vi "Logging.vi"(8 "error in (no error)":errorcluster, 11 "Node Ptr":T2 format="%.0x") -> (0 "error out":errorcluster)   [LabVIEW 2020, in "AIM MIL-STD-1553 System Explorer.lvlib" / "Implementation.lvlib"]
uses:
  Implementation.lvlib
  <vilib>/NI VeriStand/Custom Device API/Custom Device API.lvlib
  Scripting/AIM MIL-STD-1553 Scripting.lvlib
  <vilib>/NI VeriStand/Custom Device API/Custom Device Item Ref.ctl
  Shared/Data Word Format.ctl
panel:
  in  "Data Word Format":T1
  in  "Timestamp Filename":bool
  in  "File Name":string
  out "Example Log File Path":string
  in  "Enable Logging":bool
  in  "Log Directory":string
  in  "SHDocVw.IWebBrowser":refnum<k7>(container)
  in  "General Header":cluster{"Section Name":string}={"Section Name"="MIL-STD-1553 - Logging"}
  in  "Description":string
  out "Name":string
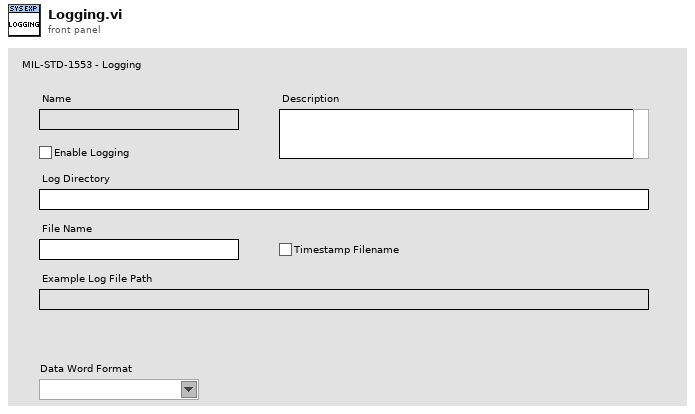
[diagram p1: front panel]
types:
  T1 = typedef "Data Word Format.ctl" = string
  T2 = typedef "Custom Device API.lvlib/Custom Device Item Ref.ctl" = u64
  T3 = typedef "Custom Device API.lvlib/Custom Device Item Info.ctl" = cluster{"Name":string, "Is Channel":bool, "GUID":string, "Is Waveform":bool}
  T4 = typedef "Custom Device API.lvlib/Custom Device Commands.ctl" = enum16{"Default", "Item renamed", "Shutdown", "Dynamic button pressed"}
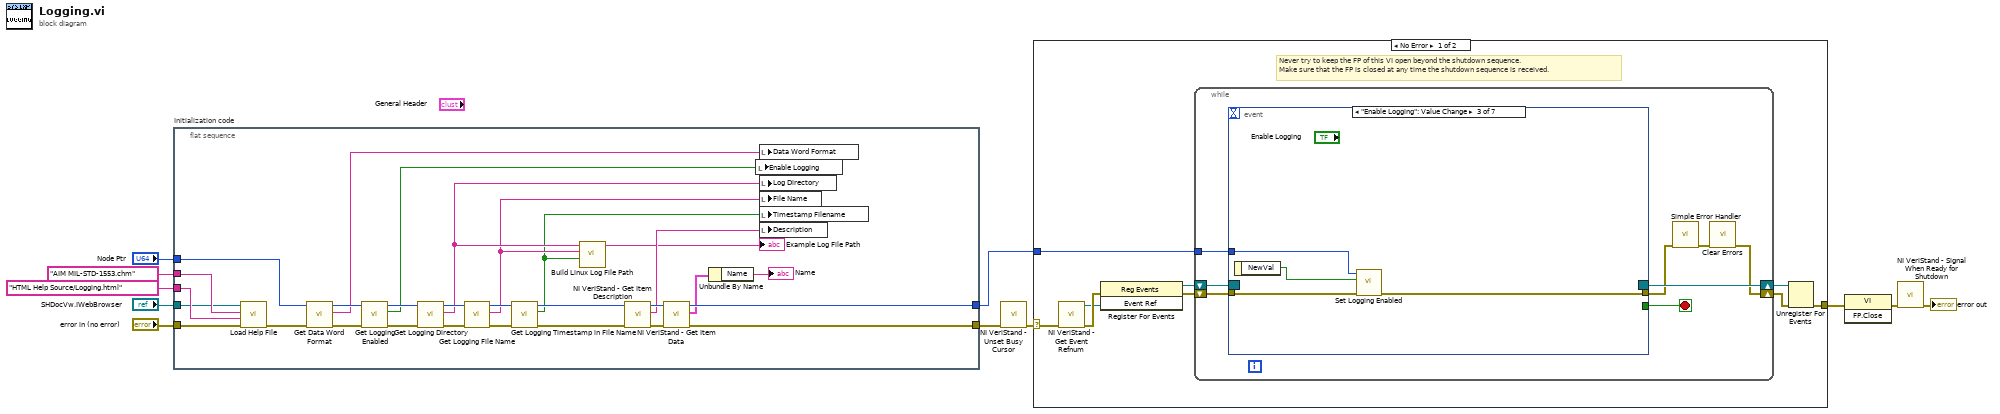
[diagram p0: block diagram]
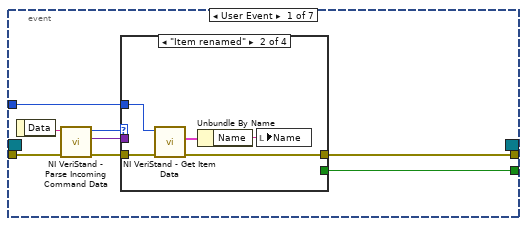
[diagram p2: hidden frame]
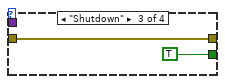
[diagram p4: hidden frame]
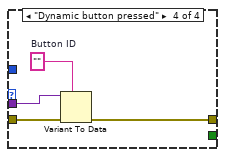
[diagram p5: hidden frame]
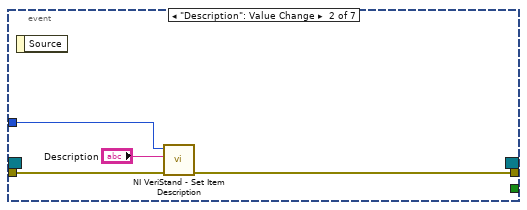
[diagram p6: hidden frame]
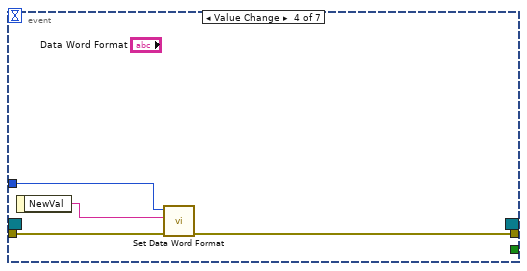
[diagram p7: hidden frame]
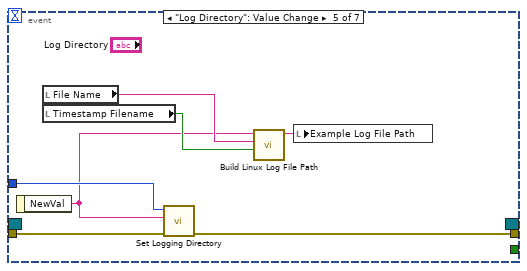
[diagram p8: hidden frame]
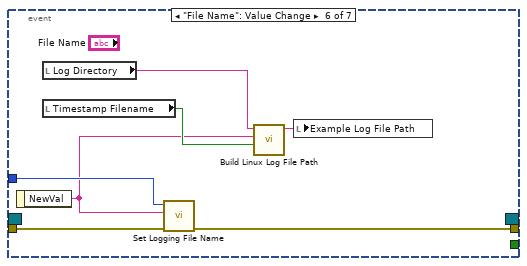
[diagram p9: hidden frame]
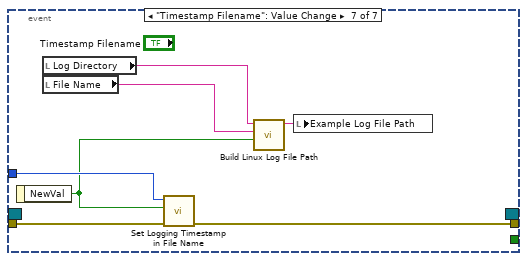
[diagram p10: hidden frame]
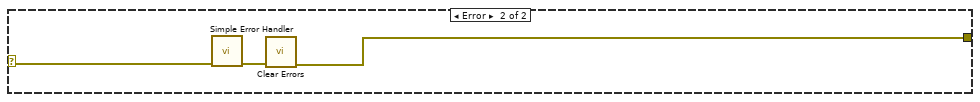
[diagram p11: hidden frame]
diagram:
  n1 = flat-sequence "Initialization code" {
    tunnel: "error in (no error)" -> [w34]
    tunnel: "Node Ptr" -> [w24]
    tunnel: [w36] -> w7
    tunnel: [w40] -> w4
    tunnel: "SHDocVw.IWebBrowser" -> [w31]
    tunnel: "HTML Help Source/Logging.html" ("CD_CHM_Section") -> [w33]
    tunnel: "AIM MIL-STD-1553.chm" ("CD_CHM_FileName") -> [w32]
    frame #0 {
      n2 = call "Load Help File.vi"("error in (no error)"=w34, "HTML File to Load"=w33, "Main CHM File"=w32, "Browser"=w31) -> ("error out"=w29:errorcluster)  [unwired: 7 in]
      n3 = call "Get Data Word Format.vi"("error in"=w29, "logging section"=w24) -> ("error out"=w25:errorcluster, "data word format"=w22:T1, "logging section out"=w23:T2)  [unwired: 7 in]
      n4 = call "Get Logging Enabled.vi"("error in"=w25, "logging section"=w23) -> ("error out"=w28:errorcluster, "logging enabled"=w26:bool, "logging section out"=w27:T2)  [unwired: 7 in]
      n5 = call "Get Logging Directory.vi"("error in"=w28, "logging section"=w27) -> ("error out"=w20:errorcluster, "directory"=w14:string, "logging section out"=w21:T2)  [unwired: 7 in]
      n6 = call "Get Logging File Name.vi"("error in"=w20, "logging section"=w21) -> ("error out"=w19:errorcluster, "file name"=w13:string, "logging section out"=w18:T2)  [unwired: 7 in]
      n7 = call "Get Logging Timestamp in File Name.vi"("error in"=w19, "logging section"=w18) -> ("error out"=w17:errorcluster, "timestamp in file name"=w12:bool, "logging section out"=w16:T2)  [unwired: 7 in]
      n8 = call "Build Linux Log File Path.vi"("Timestamp"=w12, "Name"=w13, "Log File Directory"=w14) -> ("Log File Path"=→"Example Log File Path":string)  [unwired: 7 in, 1 out]
      n9 = call <vilib>:"NI VeriStand - Get Item Description.vi"("error in (no error)"=w17, "Item Ref in"=w16) -> ("error out"=w38:errorcluster, "Description"=w35:string, "Item Ref out"=w39:T2)  [unwired: 7 out]
      n10 = call <vilib>:"NI VeriStand - Get Item Data.vi"("error in (no error)"=w38, "Item Ref in"=w39) -> ("error out"=w36:errorcluster, "Item Info"=w37:T3, "Item Ref out"=w40:T2)  [unwired: 7 out]
      n11 = Unbundle By Name(w37) -> ("Name"=→"Name":string)
      n12 = local write "Enable Logging"(w26) -> ()
      n13 = local write "Data Word Format"(w22) -> ()
      n14 = local write "Log Directory"(w14) -> ()
      n15 = local write "File Name"(w13) -> ()
      n16 = local write "Timestamp Filename"(w12) -> ()
      n17 = local write "Description"(w35) -> ()
    }
  }
  n18 = call <vilib>:"NI VeriStand - Unset Busy Cursor.vi"("error in (no error)"=w7) -> ("error out"=w6:errorcluster)  [unwired: 10 out]
  n19 = case shown="No Error" w6 {
    selector: w6 -> [w41 w113]
    tunnel: [w46 w111] -> w11
    tunnel: w4 -> [w42 _]
    frame No Error {
      # "Never try to keep the FP of this VI open beyond the shutdown sequence.\nMake sure that the FP is closed at any time the shutdown sequence is received."
      n20 = call <vilib>:"NI VeriStand - Get Event Refnum.vi"("error in (no error)"=w41) -> ("error out"=w49:errorcluster, "Event Ref"=w45:refnum<user-event>)  [unwired: 9 out]
      n21 = register-events(error in=w49, w45) -> (reference out=w43:refnum<event-registration>, error out=w44:errorcluster)  [unwired: 1 in]
      n22 = while {
        tunnel: w42 -> [w53]
        shift-right: [w50] -> w47
        shift-left: w44 -> [w56]
        shift-right: [w57] -> w48
        shift-left: w43 -> [w55]
        stop <- w54 stop-if-true
        n23 = event shown="[2] \"Enable Logging\": Value Change" {
          selector: w55 -> [_ _ _ _ _ _ _]
          dyn-events: [_ _ _ _ _ _ _] -> w57
          timeout: _ -> [_ _ _ _ _ _ _]
          tunnel: w56 -> [w65 w80 w85 w88 w96 w103 w110]
          tunnel: [w61 _ _ _ _ _ _] -> w54
          tunnel: [w60 w79 w84 w89 w94 w102 w109] -> w52
          tunnel: w53 -> [w59 w81 w83 w87 w95 w101 w108]
          event User Event {
            n24 = event-data() -> ("Data"=w64:string)  [unwired: 1 out]
            n25 = call <vilib>:"NI VeriStand - Parse Incoming Command Data.vi"("error in (no error)"=w65, "Incoming data"=w64) -> ("error out"=w63:errorcluster, "Outgoing data"=w58:variant, "Action"=w62:T4)  [unwired: 7 out]
            n26 = case shown="\"Item renamed\"" w62 {
              tunnel: w63 -> [w66 w71 w72 w77]
              tunnel: [_ _ TRUE _] -> w61
              tunnel: [w66 w68 w72 w74] -> w60
              tunnel: w59 -> [_ w70 _ _]
              tunnel: w58 -> [_ _ _ w76]
              frame "Default", Default {
              }
              frame "Item renamed" {
                n27 = call <vilib>:"NI VeriStand - Get Item Data.vi"("error in (no error)"=w71, "Item Ref in"=w70) -> ("error out"=w68:errorcluster, "Item Info"=w69:T3)  [unwired: 8 out]
                n28 = Unbundle By Name(w69) -> ("Name"=w67:string)
                n29 = local write "Name"(w67) -> ()
              }
              frame "Shutdown" {
              }
              frame "Dynamic button pressed" {
                w75 = ""  # Button ID
                n30 = Variant To Data(error in=w77, type=w75, Variant=w76) -> (error out=w74:errorcluster)  [unwired: 1 out]
              }
            }
          }
          event "Description": Value Change {
            n31 = event-data() -> ()  [unwired: 2 out]
            n32 = call <vilib>:"NI VeriStand - Set Item Description.vi"("error in (no error)"=w80, "Description"="Description", "Item Ref in"=w81) -> ("error out"=w79:errorcluster)  [unwired: 8 out]
          }
          event "Enable Logging": Value Change {
            n33 = event-data() -> ("NewVal"=w82:bool)  [unwired: 1 out]
            n34 = call "Set Logging Enabled.vi"("error in"=w85, "logging enabled"=w82, "logging section"=w83) -> ("error out"=w84:errorcluster)  [unwired: 7 in, 1 out]
          }
          event Value Change {
            n35 = event-data() -> ("NewVal"=w86:T1)  [unwired: 1 out]
            n36 = call "Set Data Word Format.vi"("error in"=w88, "data word format"=w86, "logging section"=w87) -> ("error out"=w89:errorcluster)  [unwired: 7 in, 1 out]
          }
          event "Log Directory": Value Change {
            n37 = event-data() -> ("NewVal"=w90:string)  [unwired: 1 out]
            n38 = local read "File Name"() -> (w92:string)
            n39 = local read "Timestamp Filename"() -> (w91:bool)
            n40 = call "Set Logging Directory.vi"("error in"=w96, "directory"=w90, "logging section"=w95) -> ("error out"=w94:errorcluster)  [unwired: 6 in, 1 out]
            n41 = call "Build Linux Log File Path.vi"("Timestamp"=w91, "Name"=w92, "Log File Directory"=w90) -> ("Log File Path"=w93:string)  [unwired: 7 in, 1 out]
            n42 = local write "Example Log File Path"(w93) -> ()
          }
          event "File Name": Value Change {
            n43 = event-data() -> ("NewVal"=w97:string)  [unwired: 1 out]
            n44 = local read "Log Directory"() -> (w99:string)
            n45 = local read "Timestamp Filename"() -> (w98:bool)
            n46 = call "Set Logging File Name.vi"("error in"=w103, "file name"=w97, "logging section"=w101) -> ("error out"=w102:errorcluster)  [unwired: 6 in, 1 out]
            n47 = call "Build Linux Log File Path.vi"("Timestamp"=w98, "Name"=w97, "Log File Directory"=w99) -> ("Log File Path"=w100:string)  [unwired: 7 in, 1 out]
            n48 = local write "Example Log File Path"(w100) -> ()
          }
          event "Timestamp Filename": Value Change {
            n49 = event-data() -> ("NewVal"=w106:bool)  [unwired: 1 out]
            n50 = local read "Log Directory"() -> (w105:string)
            n51 = local read "File Name"() -> (w104:string)
            n52 = call "Set Logging Timestamp in File Name.vi"("error in"=w110, "timestamp in file name"=w106, "logging section"=w108) -> ("error out"=w109:errorcluster)  [unwired: 7 in, 1 out]
            n53 = call "Build Linux Log File Path.vi"("Timestamp"=w106, "Name"=w104, "Log File Directory"=w105) -> ("Log File Path"=w107:string)  [unwired: 7 in, 1 out]
            n54 = local write "Example Log File Path"(w107) -> ()
          }
        }
        n55 = call <vilib>:"Simple Error Handler.vi"("error in (no error)"=w52) -> ("error out"=w51:errorcluster)  [unwired: 1 in, 7 out]
        n56 = call <vilib>:"Clear Errors.vi"("error in (no error)"=w51) -> ("error out"=w50:errorcluster)  [unwired: 1 in, 5 out]
      }
      n57 = Unregister For Events(event registration refnum=w48, error in=w47) -> (error out=w46:errorcluster)
    }
    frame Error {
      n58 = call <vilib>:"Simple Error Handler.vi"("error in (no error)"=w113) -> ("error out"=w112:errorcluster)  [unwired: 1 in, 7 out]
      n59 = call <vilib>:"Clear Errors.vi"("error in (no error)"=w112) -> ("error out"=w111:errorcluster)  [unwired: 1 in, 5 out]
    }
  }
  n60 = invoke class="VI" method="FP.Close"(error in=w11) -> (error out=w10:errorcluster)  [unwired: 2 in, 2 out]
  n61 = call <vilib>:"NI VeriStand - Signal When Ready for Shutdown.vi"("error in (no error)"=w10) -> ("error out"=→"error out":errorcluster)  [unwired: 10 out]
